vi "GetCreateINIFile.vi"(8 "error in (no error)":errorcluster) -> (0 "error out":errorcluster, 3 "ReportPath":path)   [LabVIEW 2014]
uses:
  <vilib>/Utility/config.llb/Write Key (Path).vi
  <vilib>/Utility/config.llb/Read Key (Path).vi
  <vilib>/Utility/config.llb/NI_LVConfig.lvlib
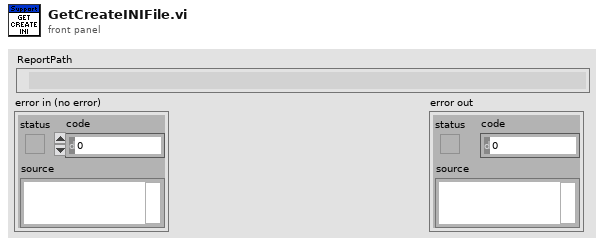
[diagram p1: front panel]
types:
  T1 = typedef "NI_LVConfig.lvlib/Config Data RefNum.ctl" = refnum<k1>
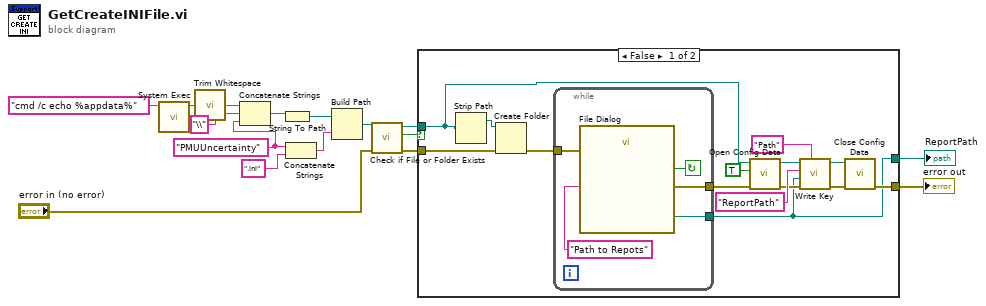
[diagram p0: block diagram]
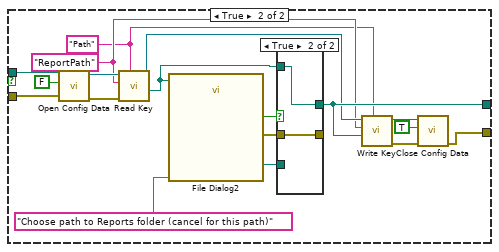
[diagram p2: hidden frame]
diagram:
  w13 = "PMUUncertainty" ("string")
  n1 = call <vilib>:"System Exec.vi"("command line"="cmd /c echo %appdata%") -> ("standard output"=w6:string)  [unwired: 7 in, 3 out]
  n2 = call <vilib>:"Trim Whitespace.vi"("string"=w6) -> ("trimmed string"=w5:string)  [unwired: 1 in]
  n3 = Concatenate Strings(w5, "\\" ("string"), w13) -> (w15:string)
  n4 = String To Path(string=w15) -> (path=w14:path)
  n5 = Concatenate Strings(w13, ".ini" ("string")) -> (w11:string)
  n6 = Build Path(base path=w14, name or relative path=w11) -> (appended path=w10:path)
  n7 = call <vilib>:"Check if File or Folder Exists.vi"("error in (no error)"="error in (no error)", "path"=w10) -> ("error out"=w4:errorcluster, "file or folder exists?"=w9:bool, "dup path"=w8:path)  [unwired: 7 in]
  n8 = case shown="False" w9 {
    tunnel: w8 -> [w19 w52]
    tunnel: w4 -> [w22 w51]
    tunnel: [w18 w36] -> w1
    tunnel: [w17 w43] -> w3
    frame False {
      n9 = Strip Path(path=w19) -> (stripped path=w20:path)  [unwired: 1 out]
      n10 = Create Folder(path (use dialog)=w20, error in=w22) -> (error out=w21:errorcluster)  [unwired: 1 in, 2 out]
      n11 = while {
        tunnel: w21 -> [w34]
        tunnel: [w32] -> w29
        tunnel: [w31] -> w17
        stop <- w33 continue-if-true
        n12 = call "File Dialog"("prompt"="Path to Repots", "error in"=w34) -> ("selected path"=w31:path, "cancelled"=w33:bool, "error out"=w32:errorcluster)  [unwired: 10 in, 1 out]
      }
      n13 = call <vilib>:"Open Config Data.vi"("error in (no error)"=w29, "create file if necessary (T)"=TRUE, "configuration file path"=w19) -> ("error out"=w26:errorcluster, "refnum"=w28:T1)  [unwired: 6 in, 1 out]
      n14 = call-poly <vilib>:"Write Key.vi"("section"="Path", "error in (no error)"=w26, "value"=w17, "key"="ReportPath", "refnum"=w28) -> ("error out"=w24:errorcluster, "refnum out"=w25:T1)  [unwired: 4 in, 1 out]
      n15 = call <vilib>:"Close Config Data.vi"("error in (no error)"=w24, "refnum"=w25) -> ("error out"=w18:errorcluster)  [unwired: 8 in, 1 out]
    }
    frame True {
      w41 = "ReportPath" ("key")
      w40 = "Path" ("section")
      n16 = call <vilib>:"Open Config Data.vi"("error in (no error)"=w51, "create file if necessary (T)"=FALSE, "configuration file path"=w52) -> ("error out"=w49:errorcluster, "refnum"=w50:T1)  [unwired: 6 in, 1 out]
      n17 = call-poly <vilib>:"Read Key.vi"("section"=w40, "error in (no error)"=w49, "key"=w41, "refnum"=w50) -> ("value"=w47:path, "refnum out"=w42:T1)  [unwired: 4 in, 2 out]
      n18 = call "File Dialog2"("start path"=w47, "prompt"="Choose path to Reports folder (cancel for this path)") -> ("selected path"=w46:path, "cancelled"=w48:bool, "error out"=w45:errorcluster)  [unwired: 10 in, 1 out]
      n19 = case shown="True" w48 {
        tunnel: w47 -> [_ w57]
        tunnel: w46 -> [w55 _]
        tunnel: [w55 w57] -> w43
        tunnel: [w54 w56] -> _
        tunnel: w45 -> [w54 w56]
        frame False {
        }
        frame True {
        }
      }
      n20 = call-poly <vilib>:"Write Key.vi"("section"=w40, "value"=w43, "key"=w41, "refnum"=w42) -> ("error out"=w38:errorcluster, "refnum out"=w39:T1)  [unwired: 5 in, 1 out]
      n21 = call <vilib>:"Close Config Data.vi"("error in (no error)"=w38, "write file if changed (T)"=TRUE, "refnum"=w39) -> ("error out"=w36:errorcluster)  [unwired: 7 in, 1 out]
    }
  }
  "ReportPath" <- w3
  "error out" <- w1
